vi "GetCellStrColor.vi"(7 "Color":u32, 8 "error in (no error)":errorcluster, 10 "Hdr Name":T1, 11 "RTD in":refnum<class "RTD.lvclass">) -> (0 "error out":errorcluster, 1 "Cell String":string, 2 "Cell Color":u32, 3 "RTD out":refnum<class "RTD.lvclass">)   [LabVIEW 2018, in "Measurement Channels.lvlib" / "RTD.lvclass"]
uses:
  RTD.lvclass
  Common/Controls/HeaderNames.ctl
  SubVIs Table/Custom Ctls Table/ge_ColType.ctl
  RTD.lvclass/RTD.ctl
  Class Channel/Channel.lvclass
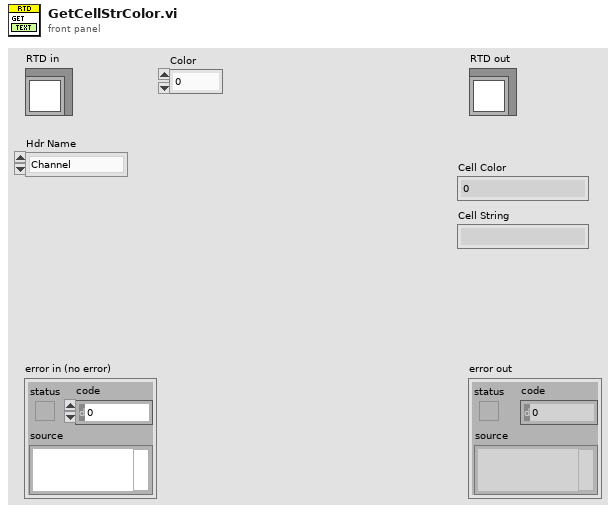
[diagram p1: front panel]
types:
  T1 = typedef "HeaderNames.ctl" = enum16{"Channel", "Device", "Spacer", "Description", "MB", "Range", "Terminal", "Coupling", "Thresh (V)", "Pulse/Rev", "Slope", "Min EU", "Min RPM", "mV/EU", "Iex", "Temp Units", "Type", "CJC Src", "CJC Val", "Ro", "Wire Cfg", "Strain Mode", "Vex", "Bridge Type", "GF", "Gauge Res", "Poisson", "Lead Res", "Init Strain", "GAF", "Scale", "Offset", "Unit (EU)", "dB?", "dB Ref", "Cal Mag", "Cal Units", "Max Temp", "Min Temp", "Max Strain", "Min Strain"}
  T2 = typedef "ge_ColType.ctl" = enum16{"Volts", "Amps", "Ohms", "TermCfg", "WireCfg", "Coup", "Slope", "Iex", "CalUnits", "ThrmUnits", "ThrmType", "CJCSrc", "BrdgType", "Strn Mode", "RTDType"}
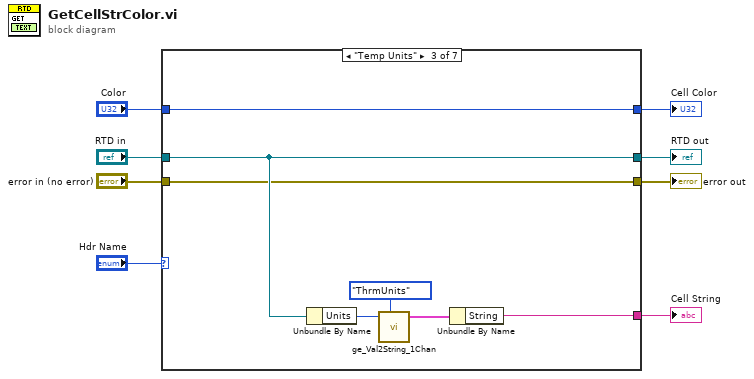
[diagram p0: block diagram]
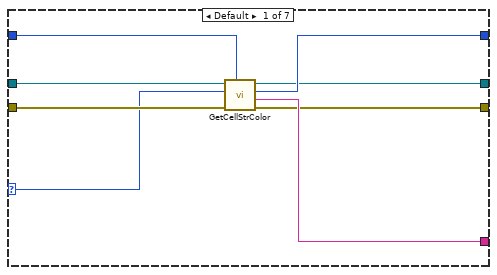
[diagram p2: hidden frame]
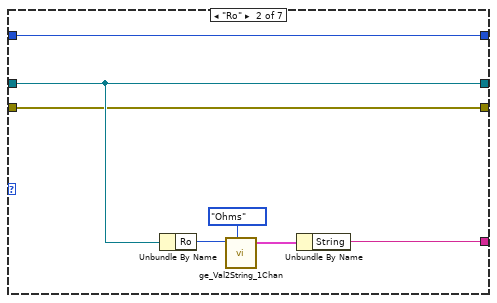
[diagram p3: hidden frame]
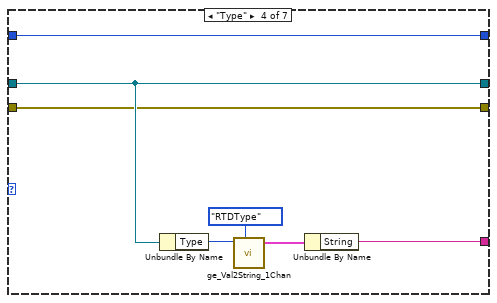
[diagram p4: hidden frame]
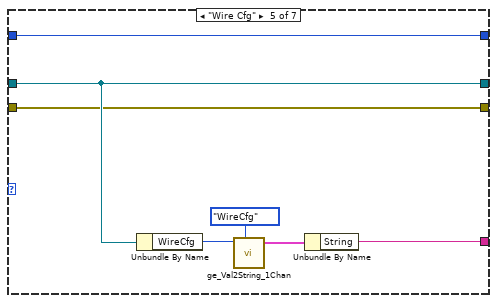
[diagram p5: hidden frame]
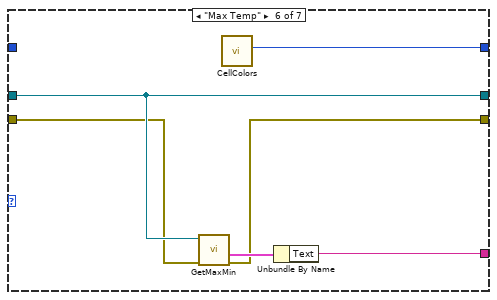
[diagram p6: hidden frame]
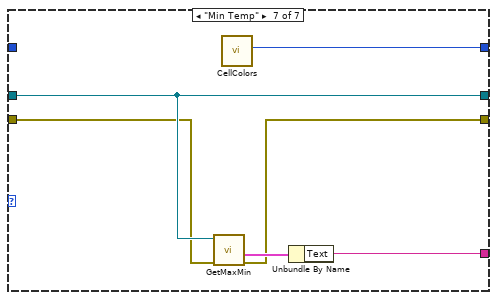
[diagram p7: hidden frame]
diagram:
  n1 = case shown="\"Temp Units\"" "Hdr Name" {
    selector: "Hdr Name" -> [w11 _ _ _ _ _ _]
    tunnel: "RTD in" -> [w9 w18 w26 w32 w39 w48 w55]
    tunnel: [w15 w21 w28 w35 w42 w47 w53] -> w1
    tunnel: [w16 w19 w27 w33 w40 w50 w56] -> w2
    tunnel: "Color" -> [w10 w19 w27 w33 w40 _ _]
    tunnel: [w14 w18 w26 w32 w39 w48 w55] -> w8
    tunnel: "error in (no error)" -> [w13 w17 w25 w31 w38 w46 w52]
    tunnel: [w12 w17 w25 w31 w38 w45 w51] -> w5
    frame Default {
      n2 = call-parent "GetCellStrColor.vi"("Color"=w10, "error in (no error)"=w13, "Hdr Name"=w11, "Channel in"=w9) -> ("error out"=w12:errorcluster, "Cell String"=w15:string, "Cell Color"=w16:u32, "Channel out"=w14:refnum<class "RTD.lvclass">)  [unwired: 4 in]
    }
    frame "Ro" {
      n3 = Unbundle By Name(w18) -> ("Ro"=w20:u16)
      n4 = call "ge_Val2String_1Chan.vi"("Value"=w20, "ColType"=ge_ColType."Ohms") -> ("String and Val"=w22:cluster{"String":string, "Value":u16})  [unwired: 5 in]
      n5 = Unbundle By Name(w22) -> ("String"=w21:string)
    }
    frame "Temp Units" {
      n6 = Unbundle By Name(w26) -> ("Units"=w24:u16)
      n7 = call "ge_Val2String_1Chan.vi"("Value"=w24, "ColType"=ge_ColType."ThrmUnits") -> ("String and Val"=w29:cluster{"String":string, "Value":u16})  [unwired: 5 in]
      n8 = Unbundle By Name(w29) -> ("String"=w28:string)
    }
    frame "Type" {
      n9 = Unbundle By Name(w32) -> ("Type"=w34:u16)
      n10 = call "ge_Val2String_1Chan.vi"("Value"=w34, "ColType"=ge_ColType."RTDType") -> ("String and Val"=w36:cluster{"String":string, "Value":u16})  [unwired: 5 in]
      n11 = Unbundle By Name(w36) -> ("String"=w35:string)
    }
    frame "Wire Cfg" {
      n12 = Unbundle By Name(w39) -> ("WireCfg"=w41:u16)
      n13 = call "ge_Val2String_1Chan.vi"("Value"=w41, "ColType"=ge_ColType."WireCfg") -> ("String and Val"=w43:cluster{"String":string, "Value":u16})  [unwired: 5 in]
      n14 = Unbundle By Name(w43) -> ("String"=w42:string)
    }
    frame "Max Temp" {
      n15 = call-dynamic "GetMaxMin.vi"("error in (no error)"=w46, "RTD in"=w48) -> ("error out"=w45:errorcluster, "Min"=w49:cluster{"Value":dbl, "Text":string})  [unwired: 6 in, 2 out]
      n16 = call "CellColors.vi"() -> ("Disabled"=w50:u32)  [unwired: 8 in, 3 out]
      n17 = Unbundle By Name(w49) -> ("Text"=w47:string)
    }
    frame "Min Temp" {
      n18 = call-dynamic "GetMaxMin.vi"("error in (no error)"=w52, "RTD in"=w55) -> ("error out"=w51:errorcluster, "Min"=w54:cluster{"Value":dbl, "Text":string})  [unwired: 6 in, 2 out]
      n19 = call "CellColors.vi"() -> ("Disabled"=w56:u32)  [unwired: 8 in, 3 out]
      n20 = Unbundle By Name(w54) -> ("Text"=w53:string)
    }
  }
  "error out" <- w5
  "RTD out" <- w8
  "Cell String" <- w1
  "Cell Color" <- w2
